vi "Read_ini_ArrayKey.vi"(8 "error in (no error)":errorcluster, 9 "key names":string[](array[string]), 10 "section":string, 11 "configuration file path":path) -> (0 "error out":errorcluster, 2 "ArrayValue":dbl[](array[numeric]))   [LabVIEW 2015]
uses:
  <vilib>/Utility/config.llb/Read Key (Double).vi
  <vilib>/Utility/config.llb/NI_LVConfig.lvlib
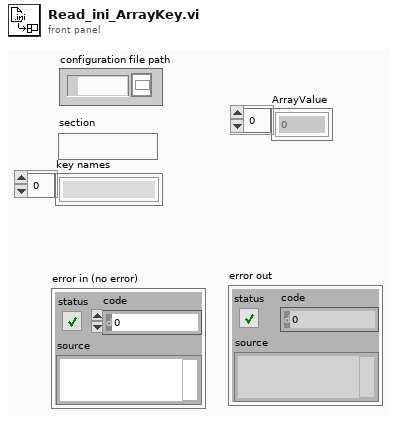
[diagram p1: front panel]
types:
  T1 = typedef "NI_LVConfig.lvlib/Config Data RefNum.ctl" = refnum<k1>
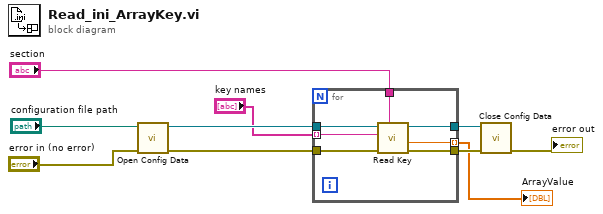
[diagram p0: block diagram]
diagram:
  n1 = call <vilib>:"Open Config Data.vi"("error in (no error)"="error in (no error)", "configuration file path"="configuration file path") -> ("error out"=w4:errorcluster, "refnum"=w3:T1)  [unwired: 7 in, 1 out]
  n2 = for {
    tunnel: [w17] -> w9
    tunnel: [w16] -> w8
    tunnel: "section" -> [w15]
    tunnel: w3 -> [w14]
    tunnel: w4 -> [w13]
    tunnel: "key names" -> [w12] mode=indexing
    tunnel: [w11] -> w1 mode=indexing
    n3 = call-poly <vilib>:"Read Key.vi"("section"=w15, "error in (no error)"=w13, "key"=w12, "refnum"=w14) -> ("error out"=w17:errorcluster, "value"=w11:dbl, "refnum out"=w16:T1)  [unwired: 4 in, 1 out]
  }
  "ArrayValue" <- w1
  n4 = call <vilib>:"Close Config Data.vi"("error in (no error)"=w9, "refnum"=w8) -> ("error out"=→"error out":errorcluster)  [unwired: 8 in, 1 out]
